vi "CompileConsoleApp.vi"(8 "error in":errorcluster, 11 "RasPi Compiler in":refnum<class "RasPi Compiler.lvclass">) -> (0 "error out":errorcluster, 3 "RasPi Compiler out":refnum<class "RasPi Compiler.lvclass">)   [LabVIEW 2014, in "RasPi Compiler.lvclass"]
uses:
  RasPi Compiler.lvclass
  RasPi Compiler.lvclass/RasPi Compiler.ctl
  Python/PythonConverter_BD/PyConvBD.lvclass
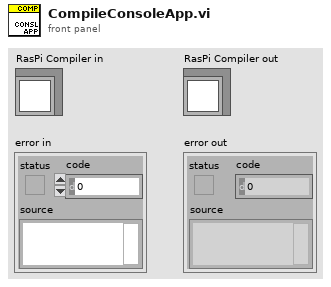
[diagram p1: front panel]
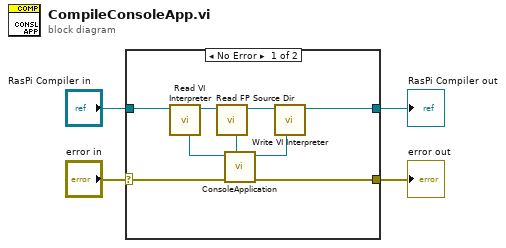
[diagram p0: block diagram]
diagram:
  n1 = case shown="No Error" "error in" {
    selector: "error in" -> [w12 w15]
    tunnel: [w11 w15] -> w3
    tunnel: [w5 w14] -> w1
    tunnel: "RasPi Compiler in" -> [w13 w14]
    frame No Error {
      n2 = call "Read VI Interpreter.vi"("RasPi Compiler in"=w13) -> ("RasPi Compiler out"=w10:refnum<class "RasPi Compiler.lvclass">, "VI Interpreter"=w8:refnum<class "VI Interpreter.lvclass">)  [unwired: 7 in]
      n3 = call "Read FP Source Dir.vi"("RasPi Compiler in"=w10) -> ("RasPi Compiler out"=w9:refnum<class "RasPi Compiler.lvclass">, "FP Source Dir"=w6:path)  [unwired: 7 in]
      n4 = call "ConsoleApplication.vi"("Source Directory"=w6, "error in"=w12, "VI Interpreter"=w8) -> ("error out"=w11:errorcluster, "VI Interpreter out"=w7:refnum<class "VI Interpreter.lvclass">)  [unwired: 5 in]
      n5 = call "Write VI Interpreter.vi"("VI Interpreter"=w7, "RasPi Compiler in"=w9) -> ("RasPi Compiler out"=w5:refnum<class "RasPi Compiler.lvclass">)  [unwired: 7 in]
    }
    frame Error {
    }
  }
  "error out" <- w3
  "RasPi Compiler out" <- w1
